vi "drotmg - Fast Givens Rotation Parameters (DBL).vi"(8 "d2 in":dbl, 9 "d1 in":dbl, 10 "y":dbl, 11 "x":dbl) -> (0 "error":i32, 1 "d2 out":dbl, 2 "d1 out":dbl, 3 "r":dbl, 4 "Rotation Matrix":T1, 5 "rotation matrix flag":i32(ring)=-1 items=["-2"=-2, "-1"=-1, "0"=0, "1"=1])   [LabVIEW 2020, in "NI_AALBLAS.lvlib"]
doc: "Calculates a fast Givens rotation matrix that zeros the <B>y</B> component of a two-element real vector and calculates the related parameters. You can use the output parameters in the drotm - Fast Givens Rotation (DBL) VI."
uses:
  <vilib>/Analysis/NI_AALBLAS.lvlib
  <vilib>/Analysis/Matrix/Datatypes/RealMatrix.ctl
  <resource>/lvblas.dll
  <vilib>/Analysis/Matrix/NI_Matrix.lvlib
panel:
  # "["
  # "]"
  # "["
  # "]"
  # "r"
  # "x"
  # "="
  # "Rotation*"
  # "0"
  # "y"
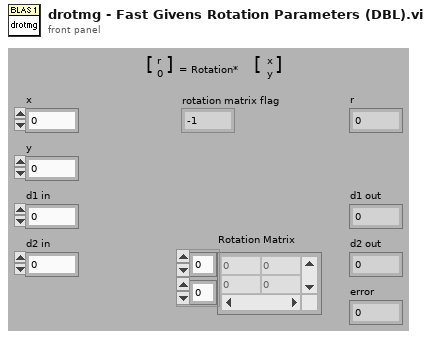
[diagram p1: front panel]
types:
  T1 = typedef "NI_Matrix.lvlib/RealMatrix.ctl" = dbl[][]
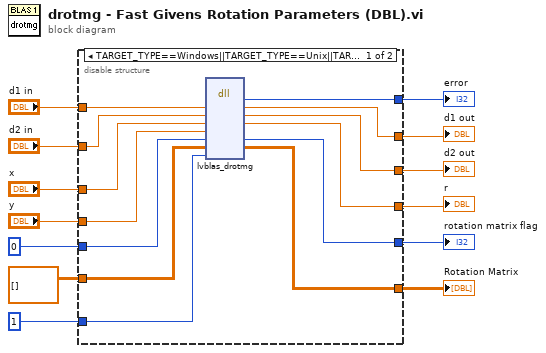
[diagram p0: block diagram]
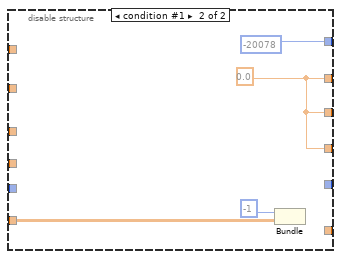
[diagram p2: hidden frame]
diagram:
  n1 = disable-structure shown="TARGET_TYPE==Windows||TARGET_TYPE==Unix||TARGET_TYPE==RT||TARGET_TYPE==Mac" {
    disable-tunnel: [w26 -20078] -> w13
    disable-tunnel: 0 -> [w25 _]
    disable-tunnel: "x" -> [w24 _]
    disable-tunnel: "y" -> [w23 _]
    disable-tunnel: "d1 in" -> [w22 _]
    disable-tunnel: "d2 in" -> [w21 _]
    disable-tunnel: [w20 w29] -> w7
    disable-tunnel: [w19 w29] -> w6
    disable-tunnel: [w18 w29] -> w5
    disable-tunnel: dbl[][] [] -> [w17 w27]
    disable-tunnel: 1 -> [w16 _]
    disable-tunnel: [w15 _] -> w2
    disable-tunnel: [w14 _] -> w1
    frame condition #0 (active) {
      n2 = dll-call lib="e:/builds/penguin/labview/branches/2020/dev/dist/resource/lvblas.*" fn="lvblas_drotmg" ("CBLAS.dll:DotProdH")("d1"=w22, "d2"=w21, "x"=w24, "y"=w23, "flag"=w25, "Rotation"=w17, "check"=w16) -> ("error"=w26:i32, "d1"=w20:dbl, "d2"=w19:dbl, "x"=w18:dbl, "flag"=w15:i32, "Rotation"=w14:dbl[][])  [unwired: 5 in, 2 out]
    }
    frame condition #1 {
      w29 = 0.0
      n3 = Bundle(-1, w27) -> ()  [unwired: 1 in, 1 out]
    }
  }
  "error" <- w13
  "d1 out" <- w7
  "d2 out" <- w6
  "r" <- w5
  "Rotation Matrix" <- w1
  "rotation matrix flag" <- w2
